vi "Circular.vi"(5 "Direction":u16(ring) items=["Clockwise", "Counter-clockwise"], 7 "Speed":dbl, 8 "error in (no error)":errorcluster, 9 "XY End":dbl[](array[numeric]), 10 "XY Center":dbl[](array[numeric]), 11 "Gantry in":refnum<class "A3200.lvclass">) -> (0 "error out":errorcluster, 3 "Gantry out":refnum<class "A3200.lvclass">)   [LabVIEW 2016, in "A3200.lvclass"]
uses:
  A3200.lvclass
  A3200.lvclass/A3200.ctl
  Drivers/Aerotech A3200/Aerotech VIs.lvlib
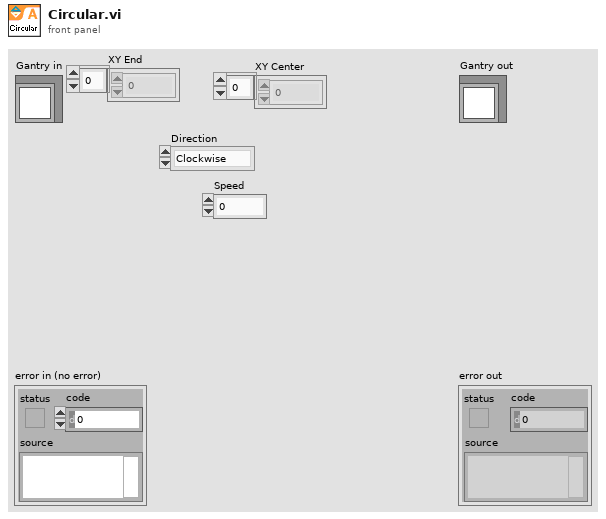
[diagram p1: front panel]
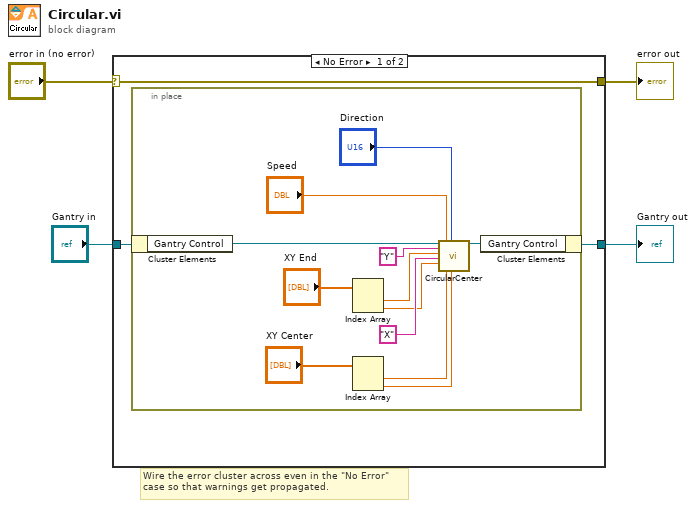
[diagram p0: block diagram]
diagram:
  # "Wire the error cluster across even in the \"No Error\"\ncase so that warnings get propagated."
  n1 = case shown="No Error" "error in (no error)" {
    selector: "error in (no error)" -> [w7 w21]
    tunnel: [w7 w21] -> w3
    tunnel: [w5 w20] -> w1
    tunnel: "Gantry in" -> [w6 w20]
    frame No Error {
      n2 = in-place {
        n3 = in-place-cluster #1(w6) -> ("Gantry Control"=w11:refnum<k24>)
        n4 = Index Array(array="XY End") -> (element #1=w13:dbl, element #2=w12:dbl)  [unwired: 2 in]
        n5 = Index Array(array="XY Center") -> (element #1=w17:dbl, element #2=w16:dbl)  [unwired: 2 in]
        n6 = call "CircularCenter.vi"("controller in"=w11, "axis 1 name"="Y", "axis 1 endpoint"=w13, "axis 2 name"="X" ("axis 1 name"), "axis 2 endpoint"=w12, "speed"="Speed", "axis 1 center point"=w17, "direction"="Direction", "axis 2 center point"=w16) -> ("controller out"=w10:refnum<k24>)  [unwired: 9 in, 1 out]
        n7 = in-place-cluster #1("Gantry Control"=w10) -> (w5:refnum<class "A3200.lvclass">)
      }
    }
    frame Error {
    }
  }
  "error out" <- w3
  "Gantry out" <- w1
